vi "Month Correction.vi"() -> (0 "Correction":i32)   [LabVIEW 2014]
panel:
  out "substring":string
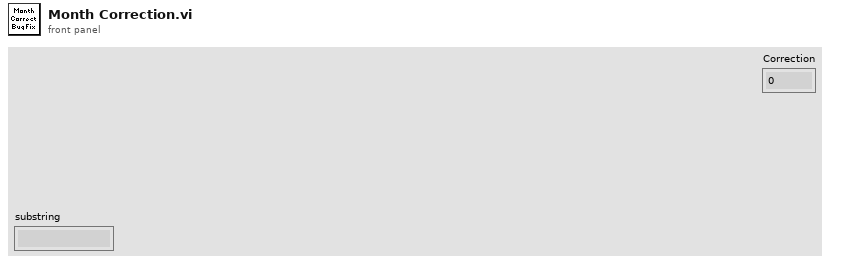
[diagram p1: front panel]
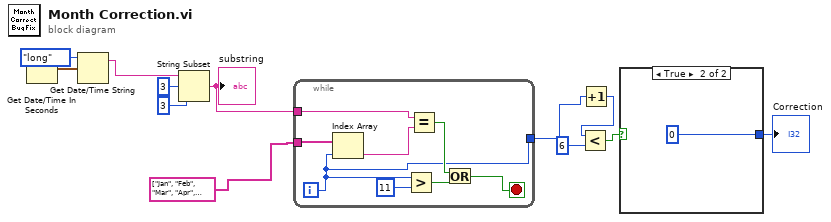
[diagram p0: block diagram]
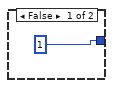
[diagram p2: hidden frame]
diagram:
  n1 = Get Date/Time In Seconds() -> (seconds since 1Jan1904=w4:timestamp)
  n2 = Get Date/Time String(date format (0)=enum16{"short", "long", "abbreviated"}."long", seconds (now)=w4) -> (date string=w3:string)  [unwired: 1 in, 1 out]
  n3 = String Subset(string=w3, offset (0)=3, length (rest)=3 ("length (rest)")) -> (substring=w9:string)
  "substring" <- w9
  n4 = while {
    tunnel: string[] ["Jan", "Feb", "Mar", "Apr", "May", "Jun", "Jul", "Aug", "Sep", "Oct", "Nov", "Dec"] ("Array") -> [w20]
    tunnel: w9 -> [w18]
    tunnel: [w13] -> w8
    i -> [w13]
    stop <- w17 stop-if-true
    n5 = Index Array(array=w20, index=w13) -> (element=w19:string)
    n6 = Greater?(x=w13, y=11) -> (0:w15:bool)
    n7 = Equal?(x=w18, y=w19) -> (x = y?=w16:bool)
    n8 = Or(x=w16, y=w15) -> (x .or. y?=w17:bool)
  }
  n9 = Increment(x=w8) -> (x+1=w6:i32)
  n10 = Less?(x=w6, y=6) -> (x < y?=w7:bool)
  n11 = case shown="True" w7 {
    tunnel: [1 ("y") 0 ("y")] -> w1
    frame False {
    }
    frame True {
    }
  }
  "Correction" <- w1
